vi "FlowControl.vi"() -> ()   [LabVIEW 2015]
uses:
  <userlib>/Fluigent/Fluigent MFCS/FluigentMFCS_Full.llb/MFCS_EZ Detect.vi
  <userlib>/Fluigent/Fluigent MFCS/FluigentMFCS_Full.llb/MFCS_EZ Initialization.vi
  <userlib>/Fluigent/Fluigent MFCS/FluigentMFCS_Full.llb/MFCS_EZ Read All Channels Pressure.vi
  <userlib>/Fluigent/Fluigent MFCS/FluigentMFCS_Full.llb/MFCS_EZ Write Channel Pressure.vi
  <userlib>/Fluigent/Fluigent MFCS/FluigentMFCS_Full.llb/MFCS_EZ Close.vi
panel:
  in  "Slide":dbl(slide) scale=0.0..10.0
  in  "stop":bool
  in  "Pressure Setpoints":dbl[](array[numeric])
  out "error out":errorcluster
  out "All Channels Pressure":dbl[](array[numeric])
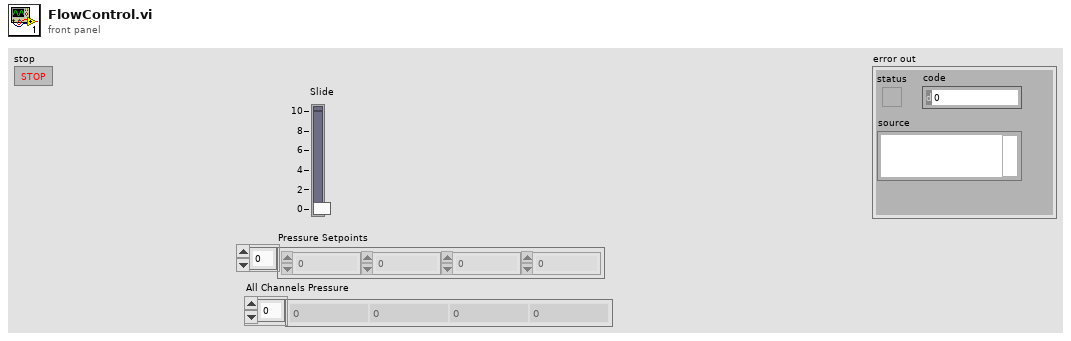
[diagram p1: front panel]
types:
  T1 = typedef "_EZmfcsSN.ctl" = u16
  T2 = typedef "_EZmfcsRefNum.ctl" = refnum<k1>
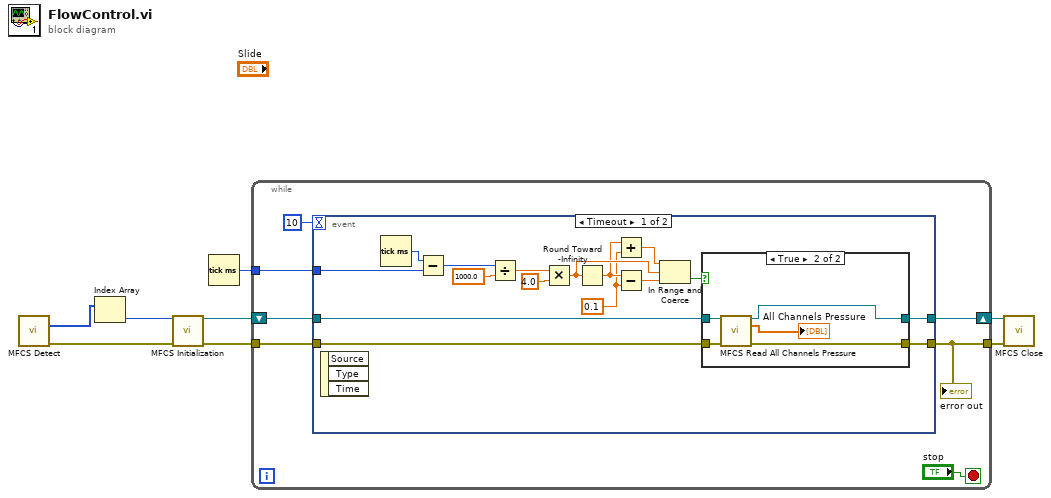
[diagram p0: block diagram]
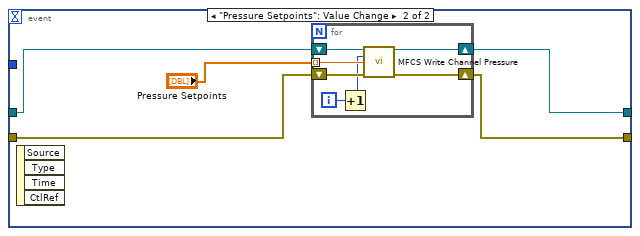
[diagram p3: hidden frame]
diagram:
  n1 = call-poly <userlib>:"MFCS Detect.vi"() -> ("[SN MFCS_EZ]"=w7:T1[], "error out"=w8:errorcluster)  [unwired: 14 in]
  n2 = Index Array(array=w7) -> (element=w6:T1)  [unwired: 1 in]
  n3 = call-poly <userlib>:"MFCS Initialization.vi"("SN MFCS_EZ"=w6, "error in (no error)"=w8) -> ("MFCS_EZ"=w4:T2, "error out"=w2:errorcluster)  [unwired: 11 in, 1 out]
  n4 = Tick Count (ms)() -> (millisecond timer value=w5:u32)
  n5 = while {
    tunnel: w5 -> [w15]
    shift-right: [w13] -> w3
    shift-left: w4 -> [w14]
    tunnel: w2 -> [w12]
    tunnel: [w9] -> w1
    stop <- "stop" stop-if-true
    n6 = event shown="[0] Timeout" {
      selector: _ -> [_ _]
      dyn-events: _ -> [_ _]
      timeout: 10 -> [_ _]
      tunnel: w15 -> [w21 _]
      tunnel: w14 -> [w26 w42]
      tunnel: [w25 w41] -> w13
      tunnel: w12 -> [w24 w40]
      tunnel: [w23 w39] -> w9
      event Timeout {
        w18 = 0.1 ("floor(x): largest int <= x")
        n7 = event-data() -> ()  [unwired: 1 in, 3 out]
        n8 = Tick Count (ms)() -> (millisecond timer value=w22:u32)
        n9 = Subtract(x=w22, y=w21) -> (x-y=w30:u32)
        n10 = Divide(x=w30, y=1000.0) -> (x/y=w29:dbl)
        n11 = Multiply(x=w29, y=4.0) -> (x*y=w20:dbl)
        n12 = Round Toward -Infinity(1:w20) -> (0:w19:dbl)
        n13 = Add(x=w19, y=w18) -> (x+y=w17:dbl)
        n14 = Subtract(x=w19, y=w18) -> (x-y=w16:dbl)
        n15 = In Range and Coerce(upper limit=w17, x=w20, lower limit=w16) -> (In Range?=w27:bool)  [unwired: 1 out]
        n16 = case shown="True" w27 {
          tunnel: w26 -> [w33 w38]
          tunnel: [w33 w37] -> w25
          tunnel: w24 -> [w32 w36]
          tunnel: [w32 w35] -> w23
          frame False {
          }
          frame True {
            n17 = call-poly <userlib>:"MFCS Read All Channels Pressure.vi"("MFCS_EZ"=w38, "error in (no error)"=w36) -> ("MFCS_EZ out"=w37:T2, "All Channels Pressure"=→"All Channels Pressure":dbl[], "error out"=w35:errorcluster)  [unwired: 11 in]
          }
        }
      }
      event "Pressure Setpoints": Value Change {
        n18 = event-data() -> ()  [unwired: 1 in, 4 out]
        n19 = for {
          tunnel: "Pressure Setpoints" -> [w50] mode=indexing
          shift-right: [w47] -> w41
          shift-left: w42 -> [w48]
          shift-right: [w45] -> w39
          shift-left: w40 -> [w46]
          i -> [w49]
          n20 = Increment(x=w49) -> (x+1=w44:i32)
          n21 = call-poly <userlib>:"MFCS Write Channel Pressure.vi"("MFCS_EZ"=w48, "Channel Number (default=1)"=w44, "Pressure (mBar)"=w50, "error in (no error)"=w46) -> ("MFCS_EZ out"=w47:T2, "error out"=w45:errorcluster)  [unwired: 10 in]
        }
      }
    }
    "error out" <- w9
  }
  n22 = call-poly <userlib>:"MFCS Close.vi"("MFCS_EZ"=w3, "error in (no error)"=w1) -> ()  [unwired: 13 in, 1 out]
